vi "SPI Configuration Main.vi"() -> ()   [LabVIEW 2014, in "SPI Configuration Tool.lvlib"]
doc: "This is the main VI for the configuration editor."
uses:
  SPI Configuration Tool.lvlib
  Controls/StateCluster.ctl
  <vilib>/NI/Configuration Framework/Repository/NISE_CEF_Repository.lvclass
  <vilib>/NI/Configuration Framework/Node/NodeRef.ctl
  <vilib>/NI/Configuration Framework/Node/NISE_CEF_Node.lvclass
  <vilib>/NI/Configuration Framework/Node/UserEventRef.ctl
  <vilib>/NI/Configuration Framework/Controls/EventCluster.ctl
  <vilib>/Utility/error.llb/DialogType.ctl
  <vilib>/NI/Configuration Framework/hierarchy repo/NISE_CEF_HierarchyRepo.lvclass
  Classes/My System/My System.lvclass
  Controls/AddMessage.ctl
  Controls/MoveMessage.ctl
  Classes/RIO Target/RIO Target.lvclass
  <vilib>/NI/AMC/Read Termination Message.vi
  <vilib>/NI/AMC/Create Single Message.vi
  <vilib>/NI/AMC/Update Message Routing Info.vi
  <vilib>/NI/AMC/Globals.vi
  <vilib>/NI/AMC/Send Message.vi
  <vilib>/NI/AMC/AMC.lvlib
  <vilib>/NI/Configuration Framework/NISE_CEF_TreeControl.lvlib
  <vilib>/NI/Configuration Framework/serializable configuration/NISE_CEF_serializable configuration.lvclass
panel:
  in  "View":string(tree)
  in  "Exit":bool
  # "SPI Inteface Generation"
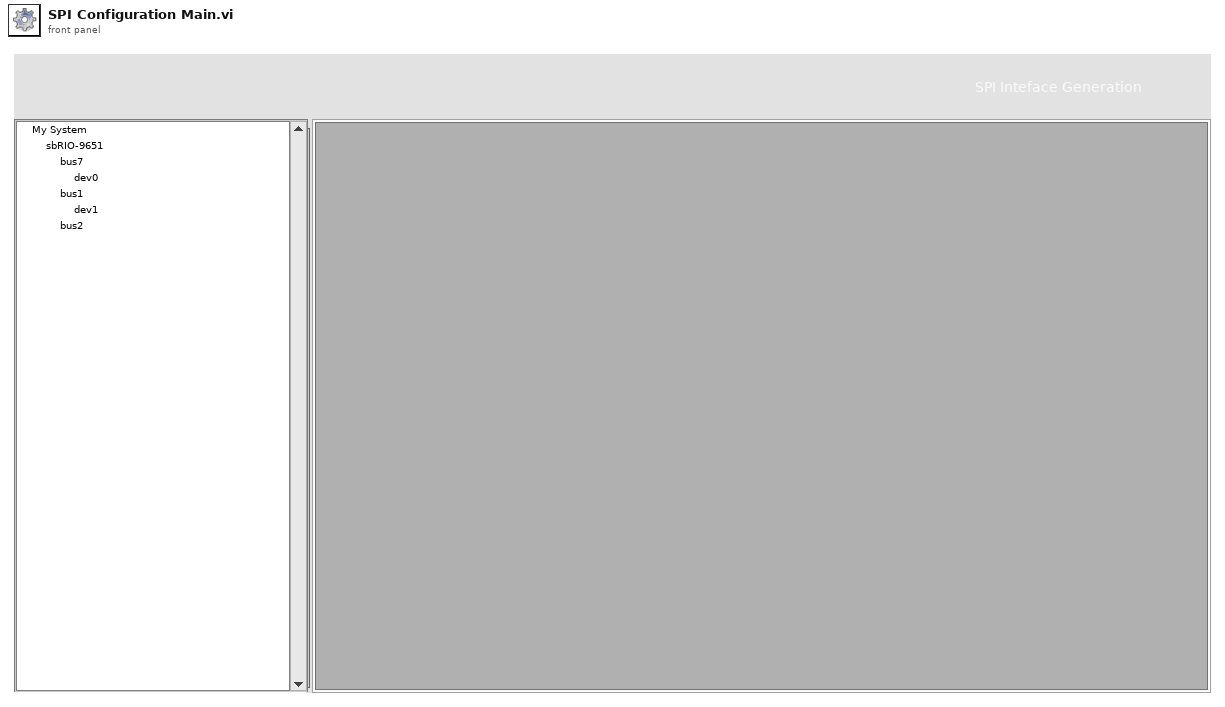
[diagram p1: front panel]
types:
  T1 = typedef "SPI Configuration Tool.lvlib/StateCluster.ctl" = cluster{"repository":refnum<class "NISE_CEF_Repository.lvclass">, "root":T2, "unsaved changes":bool, "current path":path, "user event ref":T3, "glyph path":path, "classes path":path}
  T2 = typedef "NISE_CEF_Node.lvclass/NodeRef.ctl" = refnum<data-value>
  T3 = typedef "NISE_CEF_Node.lvclass/UserEventRef.ctl" = refnum<user-event>
  T4 = typedef "AMC.lvlib/Message Queue.ctl" = refnum<queue>
  T5 = typedef "SPI Configuration Tool.lvlib/AddMessage.ctl" = cluster{"node type":string, "to add to":string}
  T6 = typedef "SPI Configuration Tool.lvlib/MoveMessage.ctl" = cluster{"node ref":T2, "new parent":T2}
  T7 = enum32{"Invalid", "Standard", "Closed", "Hidden", "Minimized", "Maximized"}
  T8 = typedef "NISE_CEF_TreeControl.lvlib/EventCluster.ctl" = cluster{"command":string, "data":string}
  T9 = typedef "SPI Configuration Tool.lvlib/FilePaths.ctl" = cluster{"glyphs":path, "classes":path}
  T10 = typedef "DialogType.ctl" = u16
  T11 = typedef "NISE_CEF_Node.lvclass/Summary.ctl" = cluster{"ID":string, "parent ID":string, "node type":string, "text":string, "additional text":string, "glyph":string, "depth":i32, "glyph overlay":string}
  T12 = typedef "LVPoint32TypeDef.ctl" = cluster{"Horizontal":i32, "Vertical":i32}
  T13 = cluster{"data name":string, "drag data":variant}[]
  T14 = typedef "NISE_CEF_Node.lvclass/NodeMenuOptions.ctl" = cluster{"removable":bool, "movable":bool, "duplicate":bool}
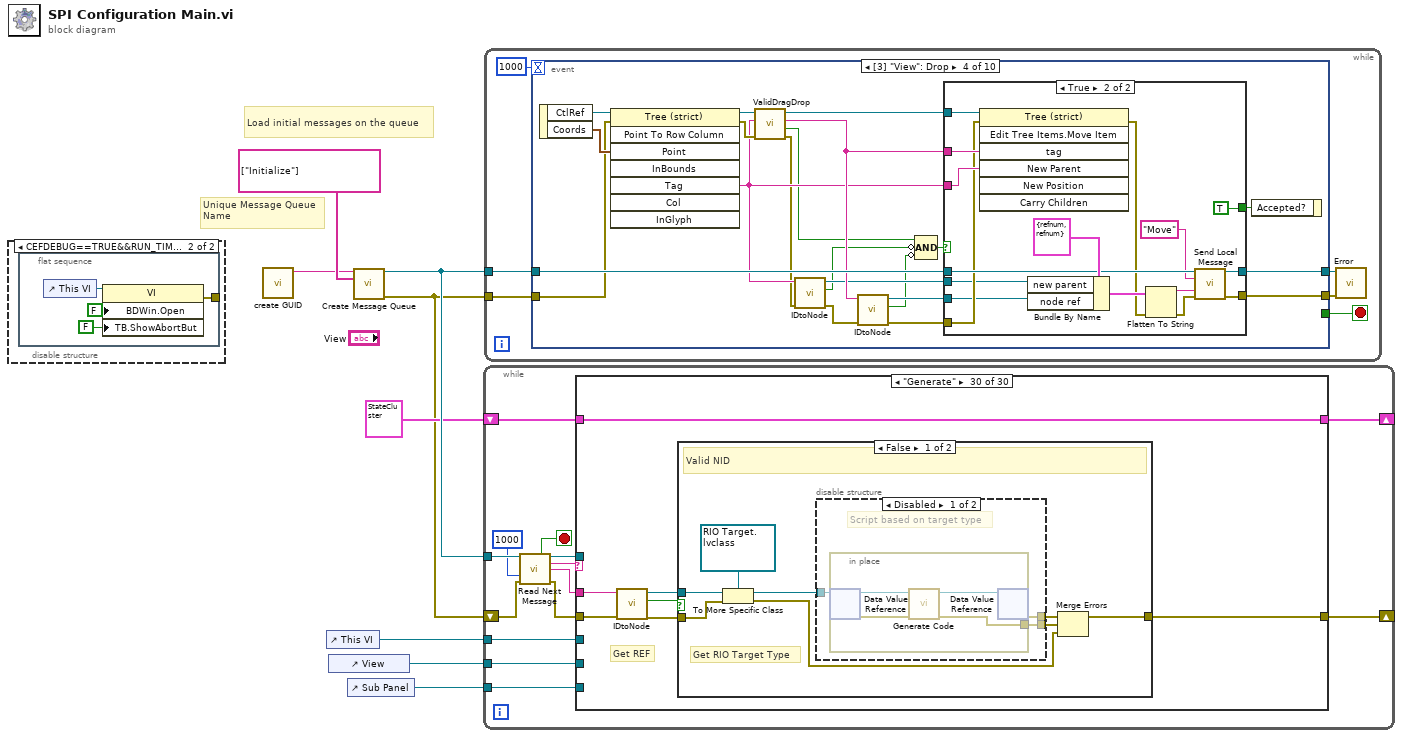
[diagram p0: block diagram]
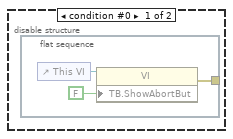
[diagram p2: hidden frame]
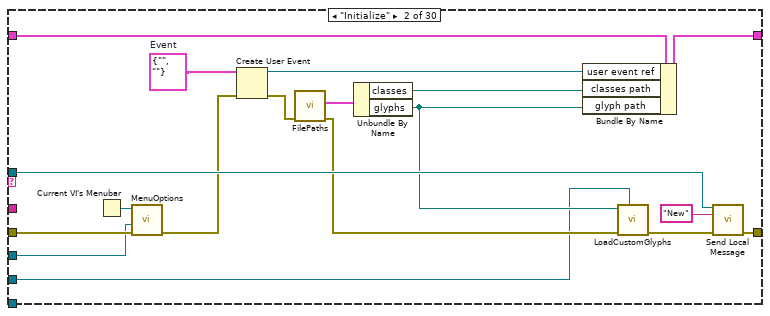
[diagram p4: hidden frame]
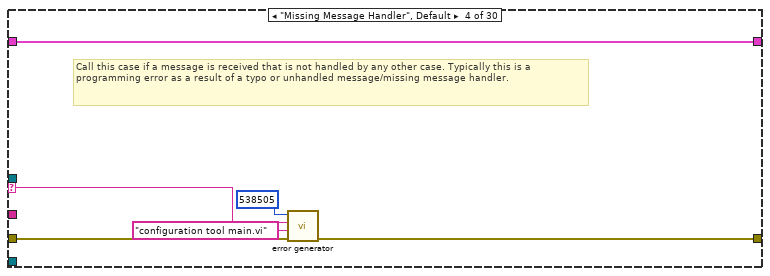
[diagram p6: hidden frame]
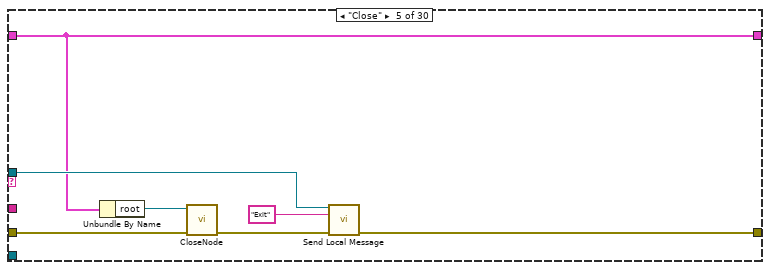
[diagram p7: hidden frame]
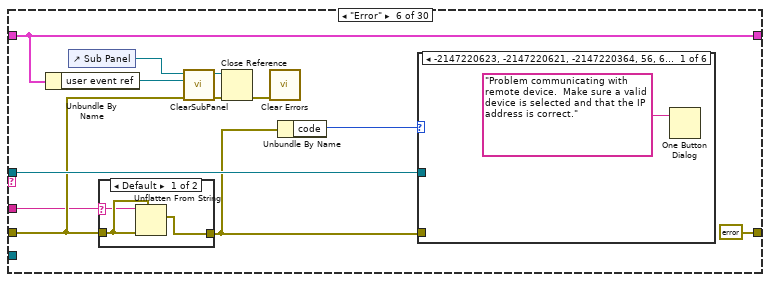
[diagram p8: hidden frame]
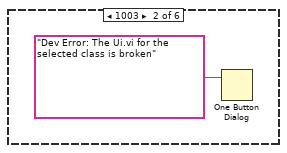
[diagram p10: hidden frame]
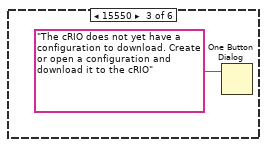
[diagram p11: hidden frame]
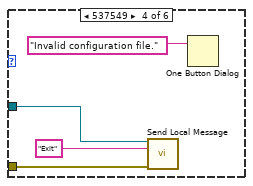
[diagram p12: hidden frame]
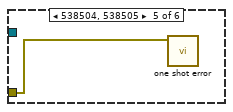
[diagram p13: hidden frame]
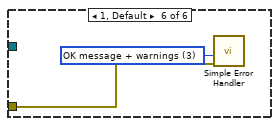
[diagram p14: hidden frame]
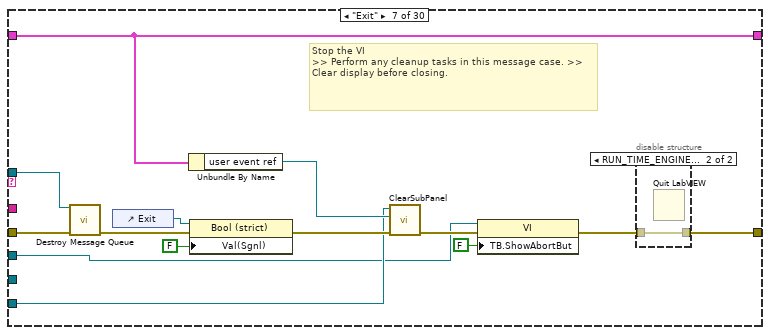
[diagram p15: hidden frame]
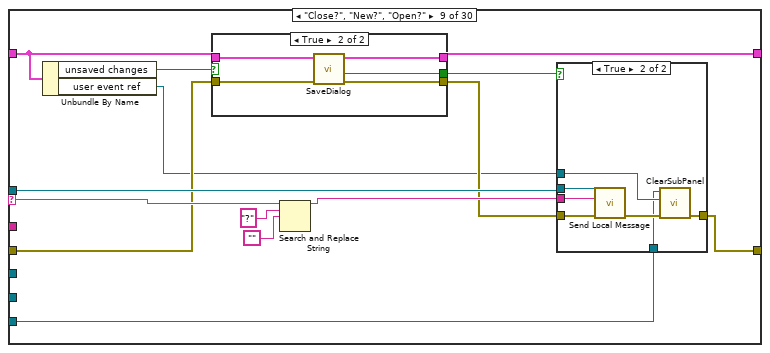
[diagram p18: hidden frame]
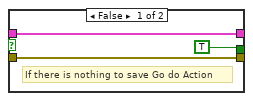
[diagram p19: hidden frame]
diagram:
  # "Unique Message Queue Name"
  # "Load initial messages on the queue"
  n1 = disable-structure shown="CEFDEBUG==TRUE&&RUN_TIME_ENGINE==False" {
    frame condition #0 {
      n2 = flat-sequence {
        tunnel: [w9] -> _
        frame #0 {
          n3 = control-ref of="This VI"() -> (w10:refnum<vi>)
          n4 = property class="VI"(reference=w10, "TB.ShowAbortBut"=FALSE ("Tool Bar:Show Abort Button")) -> (error out=w9:errorcluster)  [unwired: 1 in, 1 out]
        }
      }
    }
    frame condition #1 (active) {
      n5 = flat-sequence {
        tunnel: [w14] -> _
        frame #0 {
          n6 = control-ref of="This VI"() -> (w15:refnum<vi>)
          n7 = property class="VI"(reference=w15, "BDWin.Open"=FALSE ("Block Diagram Window:Open"), "TB.ShowAbortBut"=FALSE ("Tool Bar:Show Abort Button")) -> (error out=w14:errorcluster)  [unwired: 1 in, 1 out]
        }
      }
    }
  }
  n8 = call <vilib>:"create GUID.vi"() -> ("uuid"=w2:string)  [unwired: 10 in, 1 out]
  n9 = control-ref of="This VI"() -> (w4:refnum<vi>)
  n10 = control-ref of="View"() -> (w3:refnum<vi>)
  n11 = control-ref of="Sub Panel"() -> (w1:refnum<vi>)
  n12 = call <vilib>:"Create Message Queue.vi"("message queue name"=w2, "initial message names"=string[] ["Initialize"]) -> ("message queue out"=w7:T4, "error out"=w5:errorcluster)  [unwired: 12 in]
  n13 = while "Message Processor" {
    shift-right: [w25] -> _
    shift-left: w5 -> [w24]
    tunnel: w7 -> [w23]
    shift-right: [w21] -> _
    shift-left: T1 {"repository"=refnum, "root"=refnum, "unsaved changes"=FALSE, "current path"=path "", "user event ref"=refnum, "glyph path"=path "", "classes path"=path ""} -> [w20]
    tunnel: w4 -> [w18]
    tunnel: w3 -> [w17]
    tunnel: w1 -> [w16]
    stop <- w29 stop-if-true
    n14 = call <vilib>:"Read Next Message.vi"("message queue in"=w23, "timeout (1 ms)"=1000, "error in"=w24) -> ("exit process?"=w29:bool, "message queue out"=w19:T4, "message name"=w28:string, "message value"=w27:string, "error out"=w26:errorcluster)  [unwired: 5 in, 3 out]
    n15 = case shown="\"Generate\"" w28 {
      selector: w28 -> [_ _ _ w54 _ _ _ _ w118 _ _ _ _ _ _ _ _ _ _ w371 _ _ _ _ _ _ _ _ _ _]
      tunnel: w27 -> [_ _ _ _ _ w65 _ _ _ _ _ _ _ w240 w272 _ w300 w337 w351 w369 w411 w435 _ _ w478 w500 _ _ _ w516]
      tunnel: w26 -> [w31 w49 w51 w56 w59 w68 w104 w108 w111 w155 w166 w206 w232 w247 w273 w290 w301 w330 w350 w374 w413 w434 w459 w468 w477 w498 w503 w505 w510 w517]
      tunnel: [w31 w45 w51 w55 w63 errorcluster {"status"=FALSE, "code"=0, "source"=""} ("error out") w97 w108 w122 w146 w162 w210 w234 w244 w260 w290 w304 w321 w354 w377 w417 w431 w454 w463 w474 w493 w503 w504 w509 w512] -> w25
      tunnel: [w30 w40 w50 w57 w61 w73 w96 w107 w113 w159 w167 w213 w233 w241 w269 w289 w307 w323 w347 w378 w415 w428 w461 w467 w472 w489 w502 w507 w511 w518] -> w21
      tunnel: w20 -> [w30 w41 w50 w57 w61 w73 w96 w107 w114 w158 w168 w208 w231 w242 w270 w289 w303 w328 w355 w378 w416 w436 w461 w467 w472 w501 w502 w507 w511 w518]
      tunnel: w19 -> [_ w44 _ _ w62 w76 w103 _ w121 w160 w164 w209 _ w243 w265 _ w291 w320 _ w372 _ _ _ _ w473 w492 _ _ _ _]
      tunnel: w18 -> [_ w32 _ _ _ _ w92 _ _ _ _ _ _ _ _ _ _ _ _ _ _ _ w446 _ _ _ _ _ _ _]
      tunnel: w17 -> [_ w33 _ _ _ _ _ _ _ _ _ _ _ _ _ _ _ w324 w348 w367 w408 w429 w447 _ _ _ _ _ _ _]
      tunnel: w16 -> [_ _ _ _ _ _ w94 _ w109 _ _ _ _ _ _ _ _ _ _ _ _ _ w444 w462 w469 _ _ _ _ _]
      frame "------------Generic Operations------------" {
        # "Dummy case to add a seperation in the Case Structure menu"
      }
      frame "Initialize" {
        w35 = T8 {"command"="", "data"=""}  # Event
        n16 = Current VI's Menubar() -> (w48:refnum<k9>)
        n17 = call "MenuOptions.vi"("error in"=w49, "VI ref"=w32, "menu ref in"=w48) -> ("error out"=w39:errorcluster)  [unwired: 7 in, 1 out]
        n18 = Create User Event(user event datatype=w35, error in=w39) -> (user event=w34:refnum<user-event>, error out=w38:errorcluster)
        n19 = call "FilePaths.vi"("error in"=w38) -> ("error out"=w43:errorcluster, "paths"=w42:T9)  [unwired: 9 in]
        n20 = Unbundle By Name(w42) -> ("classes"=w37:path, "glyphs"=w36:path)
        n21 = Bundle By Name(cluster=w41, "user event ref"=w34, "classes path"=w37, "glyph path"=w36) -> (w40:T1)
        n22 = call <vilib>:"LoadCustomGlyphs.vi"("tree ref"=w33, "error in"=w43, "glyph directory"=w36) -> ("error out"=w46:errorcluster)  [unwired: 8 in]
        n23 = call <vilib>:"Send Local Message.vi"("message queue in"=w44, "message name"="New" ("Message Name"), "error in"=w46) -> ("error out"=w45:errorcluster)  [unwired: 10 in, 2 out]
      }
      frame "", "Idle" {
      }
      frame "Missing Message Handler", Default {
        # "Call this case if a message is received that is not handled by any other case. Typically this is a programming error as a result of a typo or unhandled message/missing message handler."
        n24 = call <vilib>:"error generator.vi"("error in"=w56, "source"="configuration tool main.vi", "append error message"=w54, "error code (0)"=538505) -> ("error out"=w55:errorcluster)  [unwired: 5 in]
      }
      frame "Close" {
        n25 = Unbundle By Name(w61) -> ("root"=w60:T2)
        n26 = call <vilib>:"CloseNode.vi"("error in"=w59, "node ref"=w60) -> ("error out"=w58:errorcluster)  [unwired: 9 in]
        n27 = call <vilib>:"Send Local Message.vi"("message queue in"=w62, "message name"="Exit", "error in"=w58) -> ("error out"=w63:errorcluster)  [unwired: 10 in, 2 out]
      }
      frame "Error" {
        n28 = Unbundle By Name(w73) -> ("user event ref"=w71:T3)
        n29 = control-ref of="Sub Panel"() -> (w72:refnum<vi>)
        n30 = case shown="Default" w65 {
          selector: w65 -> [w78 _]
          tunnel: w68 -> [w79 w80]
          tunnel: [w77 w80] -> w67
          frame Default {
            n31 = Unflatten From String(type=w79, binary string=w78, error in (no error)=w79) -> (value=w77:errorcluster)  [unwired: 2 in, 2 out]
          }
          frame "" {
          }
        }
        n32 = call <vilib>:"ClearSubPanel.vi"("error in"=w68, "user event ref"=w71, "sub panel ref in"=w72) -> ("error out"=w70:errorcluster, "sub panel ref out"=w69:refnum<vi>)  [unwired: 7 in]
        n33 = Close Reference(reference=w69, error in (no error)=w70) -> (error out=w66:errorcluster)
        n34 = call <vilib>:"Clear Errors.vi"("error in (no error)"=w66) -> ()  [unwired: 5 in, 2 out]
        n35 = Unbundle By Name(w67) -> ("code"=w74:i32)
        n36 = case shown="-2147220623, -2147220621, -2147220364, 56, 63" w74 {
          tunnel: w76 -> [_ _ _ w86 _ _]
          tunnel: w67 -> [_ _ _ w85 w88 w90]
          frame -2147220623, -2147220621, -2147220364, 56, 63 {
            n37 = One Button Dialog(message="Problem communicating with remote device.  Make sure a valid device is selected and that the IP address is correct.") -> ()  [unwired: 1 in, 1 out]
          }
          frame 1003 {
            n38 = One Button Dialog(message="Dev Error: The Ui.vi for the selected class is broken") -> ()  [unwired: 1 in, 1 out]
          }
          frame 15550 {
            n39 = One Button Dialog(message="The cRIO does not yet have a configuration to download. Create or open a configuration and download it to the cRIO") -> ()  [unwired: 1 in, 1 out]
          }
          frame 537549 {
            n40 = call <vilib>:"Send Local Message.vi"("message queue in"=w86, "message name"="Exit", "error in"=w85) -> ()  [unwired: 10 in, 3 out]
            n41 = One Button Dialog(message="Invalid configuration file.") -> ()  [unwired: 1 in, 1 out]
          }
          frame 538504, 538505 {
            n42 = call <vilib>:"one shot error.vi"("error in"=w88) -> ()  [unwired: 11 in]
          }
          frame 1, Default {
            w89 = T10 3 items=["no dialog", "OK message", "continue or stop message", "OK message + warnings", "continue/stop + warnings"] ("type of dialog (OK msg:1)")
            n43 = call <vilib>:"Simple Error Handler.vi"("type of dialog (OK msg:1)"=w89, "error in (no error)"=w90) -> ()  [unwired: 8 out]
          }
        }
      }
      frame "Exit" {
        # "Stop the VI                                                                             >> Perform any cleanup tasks in this message case. >> Clear display before closing."
        n44 = call <vilib>:"Destroy Message Queue.vi"("message queue in"=w103, "error in"=w104) -> ("error out"=w100:errorcluster)  [unwired: 11 in, 2 out]
        n45 = control-ref of="Exit"() -> (w102:refnum<vi>)
        n46 = Unbundle By Name(w96) -> ("user event ref"=w95:T3)
        n47 = property class="Bool (strict)"(reference=w102, error in=w100, "Val(Sgnl)"=FALSE ("Exit")) -> (error out=w99:errorcluster)  [unwired: 1 out]
        n48 = call <vilib>:"ClearSubPanel.vi"("error in"=w99, "user event ref"=w95, "sub panel ref in"=w94) -> ("error out"=w98:errorcluster)  [unwired: 7 in, 1 out]
        n49 = property class="VI"(reference=w92, error in=w98, "TB.ShowAbortBut"=FALSE ("Tool Bar:Show Abort Button")) -> (error out=w93:errorcluster)  [unwired: 1 out]
        n50 = disable-structure shown="RUN_TIME_ENGINE==True" {
          disable-tunnel: [w105 w106] -> w97
          disable-tunnel: w93 -> [w105 w106]
          frame condition #0 (active) {
          }
          frame condition #1 {
            n51 = Quit LabVIEW() -> ()  [unwired: 1 in]
          }
        }
      }
      frame "------------Menu Operations--------------" {
        # "Dummy case to add a seperation in the Case Structure menu"
      }
      frame "Close?", "New?", "Open?" {
        n52 = Unbundle By Name(w114) -> ("unsaved changes"=w116:bool, "user event ref"=w110:T3)
        n53 = case shown="True" w116 {
          tunnel: [TRUE ("SaveFlag") w130] -> w115
          tunnel: w114 -> [w124 w129]
          tunnel: [w124 w128] -> w113
          tunnel: w111 -> [w123 w127]
          tunnel: [w123 w126] -> w112
          frame False {
            # "If there is nothing to save Go do Action"
          }
          frame True {
            n54 = call "SaveDialog.vi"("error in"=w127, "state in"=w129) -> ("error out"=w126:errorcluster, "new"=w130:bool, "state out"=w128:T1)  [unwired: 7 in]
          }
        }
        n55 = Search and Replace String(input string=w118, search string="?", replace string="") -> (result string=w117:string)  [unwired: 5 in, 3 out]
        n56 = case shown="True" w115 {
          tunnel: w112 -> [w131 w138]
          tunnel: [w131 w134] -> w122
          tunnel: w121 -> [_ w137]
          tunnel: w117 -> [_ w136]
          tunnel: w110 -> [_ w133]
          tunnel: w109 -> [_ w132]
          frame False {
          }
          frame True {
            n57 = call <vilib>:"Send Local Message.vi"("message queue in"=w137, "message name"=w136, "error in"=w138) -> ("error out"=w135:errorcluster)  [unwired: 10 in, 2 out]
            n58 = call <vilib>:"ClearSubPanel.vi"("error in"=w135, "user event ref"=w133, "sub panel ref in"=w132) -> ("error out"=w134:errorcluster)  [unwired: 7 in, 1 out]
          }
        }
      }
      frame "New" {
        n59 = Unbundle By Name(w158) -> ("classes path"=w157:path)
        n60 = call-dynamic "Initialize.vi"("error in"=w155, "path"=w157, "repository in"=refnum<class "NISE_CEF_HierarchyRepo.lvclass"> refnum ("NISE_CEF_HierarchyRepo.lvclass")) -> ("error out"=w156:errorcluster, "repository out"=w149:refnum<class "NISE_CEF_HierarchyRepo.lvclass">)  [unwired: 7 in]
        n61 = call-dynamic "Initialize.vi"("error in"=w156, "node in"=refnum<class "My System.lvclass"> refnum ("My System.lvclass")) -> ("error out"=w143:errorcluster, "data value reference"=w144:T2)  [unwired: 7 in, 1 out]
        n62 = call <vilib>:"NodetoID.vi"("error in"=w143, "node ref"=w144) -> ("error out"=w142:errorcluster, "ID"=w140:string)  [unwired: 8 in]
        n63 = call <vilib>:"Send Local Message.vi"("message queue in"=w160, "message name"="PopulateTree", "error in"=w142) -> ("message queue out"=w145:T4, "error out"=w151:errorcluster)  [unwired: 10 in, 1 out]
        n64 = Current VI's Menubar() -> (w150:refnum<k9>)
        n65 = call <vilib>:"NewMenu.vi"("error in"=w151, "menu ref in"=w150, "NISE_CEF_Repository in"=w149) -> ("error out"=w147:errorcluster, "NISE_CEF_Repository out"=w148:refnum<class "NISE_CEF_HierarchyRepo.lvclass">)  [unwired: 6 in, 1 out]
        n66 = Bundle By Name(cluster=w158, "current path"=path "", "unsaved changes"=FALSE, "repository"=w148, "root"=w144) -> (w159:T1)
        n67 = call <vilib>:"Send Local Message.vi"("message queue in"=w145, "message name"="ActivateNode", "message value"=w140, "error in"=w147) -> ("error out"=w146:errorcluster)  [unwired: 9 in, 2 out]
      }
      frame "Open" {
        n68 = in-place {
          in-place-border: w166 -> [w174]
          in-place-border: [w173] -> w163
          n69 = in-place-cluster #1(w168) -> ("current path"=w170:path, "repository"=w182:refnum<class "NISE_CEF_Repository.lvclass">, "root"=w178:T2)  [unwired: 1 out]
          n70 = call "generate default path.vi"("current file path"=w170) -> ("browse path"=w169:path)  [unwired: 10 in]
          n71 = call "FileDialog.vi"("error in"=w174, "start path"=w169) -> ("error out"=w175:errorcluster, "cancelled"=w176:bool, "selected path"=w172:path)  [unwired: 7 in]
          n72 = Compound Arithmetic op=OR(invert w176) -> (w177:bool)
          n73 = case shown="True" w177 {
            tunnel: w182 -> [w183 w195]
            tunnel: [w183 w193] -> w180
            tunnel: [w184 w191] -> w173
            tunnel: [w185 w190] -> w179
            tunnel: w172 -> [_ w188]
            tunnel: w175 -> [w184 w187]
            tunnel: w178 -> [w185 w186]
            frame False {
            }
            frame True {
              n74 = call-dynamic "Open.vi"("error in"=w187, "file path"=w188, "repository in"=w195) -> ("error out"=w192:errorcluster, "invalid?"=w189:bool, "repository out"=w194:refnum<class "NISE_CEF_Repository.lvclass">)  [unwired: 6 in]
              n75 = case shown="False" w189 {
                tunnel: w194 -> [w200 w203]
                tunnel: [w199 w203] -> w193
                tunnel: w192 -> [w198 w202]
                tunnel: [w197 w202] -> w191
                tunnel: [w196 w201] -> w190
                tunnel: w186 -> [_ w201]
                frame False {
                  n76 = call-dynamic "WriteTree.vi"("error in"=w198, "repository in"=w200) -> ("error out"=w197:errorcluster, "root"=w196:T2, "repository out"=w199:refnum<class "NISE_CEF_Repository.lvclass">)  [unwired: 7 in]
                }
                frame True {
                }
              }
            }
          }
          n77 = Select(t=w170, s=w173, f=w172) -> (s? t:f=w171:path)
          n78 = in-place-cluster #1("current path"=w171, "unsaved changes"=FALSE ("SaveFlag"), "repository"=w180, "root"=w179) -> (w167:T1)
        }
        n79 = call <vilib>:"Send Local Message.vi"("message queue in"=w164, "message name"="PopulateTree", "error in"=w163) -> ("error out"=w162:errorcluster)  [unwired: 10 in, 2 out]
      }
      frame "Save" {
        n80 = in-place {
          in-place-border: w206 -> [w218]
          in-place-border: [w217] -> w205
          in-place-border: [w215] -> w204
          n81 = in-place-cluster #2(w208) -> ("current path"=w216:path, "root"=w219:T2, "repository"=w220:refnum<class "NISE_CEF_Repository.lvclass">)
          n82 = Empty String/Path?(string/path=w216) -> (empty?=w215:bool)
          n83 = call-dynamic "ReadTree.vi"("error in"=w218, "root"=w219, "repository in"=w220) -> ("error out"=w217:errorcluster, "repository out"=w214:refnum<class "NISE_CEF_Repository.lvclass">)  [unwired: 7 in]
          n84 = in-place-cluster #2("current path"=w216, "root"=w219, "repository"=w214) -> (w207:T1)
        }
        n85 = case shown="True" w204 {
          tunnel: w207 -> [w224 w226]
          tunnel: [w223 w225] -> w213
          tunnel: [w222 w227] -> w211
          tunnel: w205 -> [w221 w228]
          frame False {
            n86 = call "Save.vi"("error in"=w221, "state in"=w224) -> ("error out"=w222:errorcluster, "state out"=w223:T1)  [unwired: 8 in]
          }
          frame True {
            # "Empty path use Dialog"
            n87 = call "SaveAs.vi"("error in"=w228, "state in"=w226) -> ("error out"=w227:errorcluster, "state out"=w225:T1)  [unwired: 7 in, 1 out]
          }
        }
        n88 = call <vilib>:"Send Local Message.vi"("message queue in"=w209, "message name"="PopulateTree", "error in"=w211) -> ("error out"=w210:errorcluster)  [unwired: 10 in, 2 out]
      }
      frame "SaveAs" {
        n89 = in-place {
          in-place-border: w232 -> [w236]
          in-place-border: [w235] -> w230
          n90 = in-place-cluster #3(w231) -> ("root"=w237:T2, "repository"=w239:refnum<class "NISE_CEF_Repository.lvclass">)
          n91 = call-dynamic "ReadTree.vi"("error in"=w236, "root"=w237, "repository in"=w239) -> ("error out"=w235:errorcluster, "repository out"=w238:refnum<class "NISE_CEF_Repository.lvclass">)  [unwired: 7 in]
          n92 = in-place-cluster #3("root"=w237, "repository"=w238) -> (w229:T1)
        }
        n93 = call "SaveAs.vi"("error in"=w230, "state in"=w229) -> ("error out"=w234:errorcluster, "state out"=w233:T1)  [unwired: 7 in, 1 out]
      }
      frame "Custom View" {
        n94 = in-place {
          in-place-border: w247 -> [w258]
          in-place-border: [w257] -> w245
          in-place-border: w240 -> [w248]
          n95 = in-place-cluster #4(w242) -> ("repository"=w252:refnum<class "NISE_CEF_Repository.lvclass">, "root"=w251:T2)
          n96 = call-dynamic "ReadTree.vi"("error in"=w258, "root"=w251, "repository in"=w252) -> ("error out"=w255:errorcluster, "repository out"=w254:refnum<class "NISE_CEF_Repository.lvclass">)  [unwired: 7 in]
          n97 = call-dynamic "CustomView.vi"("error in"=w255, "view name"=w248, "repository in"=w254) -> ("error out"=w256:errorcluster, "repository out"=w253:refnum<class "NISE_CEF_Repository.lvclass">)  [unwired: 7 in]
          n98 = call-dynamic "WriteTree.vi"("error in"=w256, "repository in"=w253) -> ("error out"=w257:errorcluster, "root"=w249:T2, "repository out"=w250:refnum<class "NISE_CEF_Repository.lvclass">)  [unwired: 7 in]
          n99 = in-place-cluster #4("repository"=w250, "root"=w249) -> (w241:T1)
        }
        n100 = call <vilib>:"Send Local Message.vi"("message queue in"=w243, "message name"="PopulateTree", "error in"=w245) -> ("error out"=w244:errorcluster)  [unwired: 10 in, 2 out]
      }
      frame "CustomFileMenu" {
        n101 = Unflatten From String(type=cluster{"ItemTag":string, string} {"ItemTag"="", ""} ("output cluster"), binary string=w272, error in (no error)=w273) -> (value=w259:cluster{"ItemTag":string, string}, error out=w268:errorcluster)  [unwired: 2 in, 1 out]
        n102 = Unbundle By Name(w270) -> ("repository"=w267:refnum<class "NISE_CEF_Repository.lvclass">)
        n103 = Unbundle(w259) -> ("ItemTag"=w264:string, w263:string)
        n104 = call-dynamic "HandleMenu.vi"("message queue"=w265, "error in"=w268, "Item Path"=w263, "ItemTag"=w264, "NISE_CEF_Repository in"=w267) -> ("error out"=w262:errorcluster, "handled?"=w261:bool, "NISE_CEF_Repository out"=w266:refnum<class "NISE_CEF_Repository.lvclass">)  [unwired: 4 in]
        n105 = case shown="False" w261 {
          tunnel: w262 -> [w277 w288]
          tunnel: [w278 w288] -> w260
          tunnel: w259 -> [w276 _]
          frame False {
            n106 = Unbundle(w276) -> ("ItemTag"=w275:string, w274:string)
            n107 = disable-structure shown="Default" {
              disable-tunnel: w277 -> [w284 w287]
              disable-tunnel: [w283 w287] -> w278
              disable-tunnel: w274 -> [w282 _]
              disable-tunnel: w275 -> [w281 _]
              frame condition #0 (active) {
                n108 = Concatenate Strings(w281, "::" ("string"), w282) -> (w280:string)
                n109 = call <vilib>:"error generator.vi"("error in"=w284, "source"="configuration tool main.vi", "append error message"=w280, "error code (0)"=538506) -> ("error out"=w283:errorcluster)  [unwired: 5 in]
              }
              frame condition #1 {
              }
            }
          }
          frame True {
          }
        }
        n110 = Bundle By Name(cluster=w270, "repository"=w266) -> (w269:T1)
      }
      frame "-------TreeControl Operations-----------" {
        # "Dummy case to add a seperation in the Case Structure menu"
      }
      frame "Select Target" {
        n111 = in-place {
          in-place-border: w301 -> [w311]
          in-place-border: w300 -> [w310]
          in-place-border: [w309] -> w297
          in-place-border: [w308] -> w298
          n112 = in-place-cluster #5(w303) -> ("repository"=w313:refnum<class "NISE_CEF_Repository.lvclass">)
          n113 = call-dynamic "GetClassPath.vi"("error in"=w311, "class name"=w310, "Repository in"=w313) -> ("error out"=w309:errorcluster, "class path"=w308:path, "Repository out"=w312:refnum<class "NISE_CEF_Repository.lvclass">)  [unwired: 6 in]
          n114 = in-place-cluster #5("repository"=w312) -> (w302:T1)
        }
        n115 = call <vilib>:"Get LV Class Default Value.vi"("error in (no error)"=w297, "class path"=w298) -> ("error out"=w296:errorcluster, "object"=w299:refnum<class>)  [unwired: 8 in]
        n116 = To More Specific Class(target class=refnum<class "NISE_CEF_Node.lvclass"> refnum ("Node.lvclass"), reference=w299, error in=w296) -> (specific class reference=w294:refnum<class "NISE_CEF_Node.lvclass">, error out=w293:errorcluster)
        n117 = call-dynamic "Initialize.vi"("error in"=w293, "node in"=w294) -> ("error out"=w292:errorcluster, "data value reference"=w306:T2)  [unwired: 7 in, 1 out]
        n118 = Bundle By Name(cluster=w302, "root"=w306) -> (w307:T1)
        n119 = call <vilib>:"Send Local Message.vi"("message queue in"=w291, "message name"="PopulateTree", "error in"=w292) -> ("error out"=w304:errorcluster)  [unwired: 10 in, 2 out]
      }
      frame "AddNode" {
        n120 = Unflatten From String(type=T5 {"node type"="", "to add to"=""} ("input cluster"), binary string=w337) -> (value=w335:T5)  [unwired: 3 in, 2 out]
        n121 = Unbundle By Name(w335) -> ("to add to"=w333:string, "node type"=w326:string)
        n122 = in-place {
          in-place-border: w330 -> [w343]
          in-place-border: [w342] -> w329
          in-place-border: w326 -> [w341]
          in-place-border: [w340] -> w325
          n123 = in-place-cluster #6(w328) -> ("repository"=w345:refnum<class "NISE_CEF_Repository.lvclass">)
          n124 = call-dynamic "GetClassPath.vi"("error in"=w343, "class name"=w341, "Repository in"=w345) -> ("error out"=w342:errorcluster, "class path"=w340:path, "Repository out"=w344:refnum<class "NISE_CEF_Repository.lvclass">)  [unwired: 6 in]
          n125 = in-place-cluster #6("repository"=w344) -> (w327:T1)
        }
        n126 = call <vilib>:"Get LV Class Default Value.vi"("error in (no error)"=w329, "class path"=w325) -> ("error out"=w338:errorcluster, "object"=w339:refnum<class>)  [unwired: 8 in]
        n127 = To More Specific Class(target class=refnum<class "NISE_CEF_Node.lvclass"> refnum ("Node.lvclass"), reference=w339, error in=w338) -> (specific class reference=w318:refnum<class "NISE_CEF_Node.lvclass">, error out=w332:errorcluster)
        n128 = call <vilib>:"AddNode.vi"("error in"=w332, "node in"=w318, "parent node ID"=w333) -> ("error out"=w331:errorcluster, "summary"=w316:T11[])  [unwired: 7 in]
        n129 = Index Array(array=w316) -> (element=w315:T11)  [unwired: 1 in]
        n130 = call <vilib>:"PopulateTreeSumary.vi"("error in"=w331, "array"=w316, "tree ref in"=w324) -> ("error out"=w317:errorcluster)  [unwired: 8 in]
        n131 = Bundle By Name(cluster=w327, "unsaved changes"=TRUE) -> (w323:T1)
        n132 = Unbundle By Name(w315) -> ("ID"=w314:string)
        n133 = call <vilib>:"Send Local Message.vi"("message queue in"=w320, "message name"="ActivateNode", "message value"=w314, "error in"=w317) -> ("error out"=w321:errorcluster)  [unwired: 9 in, 2 out]
        n134 = property on="View" class="Tree (strict)"("Value"=w314) -> ()  [unwired: 2 in, 2 out]
      }
      frame "Duplicate" {
        n135 = call <vilib>:"IDtoNode.vi"("error in"=w350, "ID"=w351) -> ("error out"=w352:errorcluster, "invalid Id"=w349:bool, "node ref"=w353:T2)  [unwired: 7 in]
        n136 = case shown="False" w349 {
          tunnel: [w364 w365] -> w354
          tunnel: w353 -> [w363 _]
          tunnel: w352 -> [w360 w365]
          tunnel: w348 -> [w356 _]
          frame False {
            n137 = call <vilib>:"DuplicateNode.vi"("same parent?"=TRUE ("s"), "error in"=w360, "node ref in"=w363) -> ("error out"=w361:errorcluster, "new node ref"=w362:T2)  [unwired: 7 in]
            n138 = call <vilib>:"Summary.vi"("error in"=w361, "node self ref"=w362) -> ("error out"=w358:errorcluster, "summary"=w357:T11[])  [unwired: 8 in]
            n139 = call <vilib>:"PopulateTreeSumary.vi"("error in"=w358, "array"=w357, "tree ref in"=w356) -> ("error out"=w364:errorcluster)  [unwired: 8 in]
          }
          frame True {
          }
        }
        n140 = Bundle By Name(cluster=w355, "unsaved changes"=TRUE) -> (w347:T1)
      }
      frame "CustomMenuAction" {
        # "Pass NID into parameters\nto use in other cases"
        n141 = Match Pattern(string=w369, regular expression=":") -> (before substring=w368:string, after substring=w366:string)  [unwired: 1 in, 2 out]
        n142 = call <vilib>:"IDtoNode.vi"("error in"=w374, "ID"=w366) -> ("error out"=w375:errorcluster, "invalid Id"=w373:bool, "node ref"=w376:T2)  [unwired: 7 in]
        n143 = case shown="False" w373 {
          tunnel: [w383 w407] -> w377
          tunnel: w376 -> [w379 _]
          tunnel: w375 -> [w386 w407]
          tunnel: w372 -> [w387 _]
          tunnel: w371 -> [_ _]
          tunnel: w368 -> [w384 _]
          tunnel: w367 -> [w381 _]
          tunnel: w366 -> [w380 _]
          frame False {
            n144 = in-place {
              in-place-border: w387 -> [w405]
              in-place-border: w386 -> [w403]
              in-place-border: [w402] -> w382
              in-place-border: [w401] -> w385
              in-place-border: w384 -> [w400]
              in-place-border: w381 -> [w399]
              in-place-border: w380 -> [w398]
              n145 = in-place-dvr #7(w379) -> (w406:refnum<class "NISE_CEF_Node.lvclass">)  [unwired: 1 out]
              n146 = call-dynamic "MenuHandler.vi"("tree control"=w399, "main message queue"=w405, "error in"=w403, "parameters"=w398, "menu string"=w400, "NISE_CEF_Node in"=w406) -> ("error out"=w402:errorcluster, "Unhandled"=w401:bool, "NISE_CEF_Node out"=w404:refnum<class "NISE_CEF_Node.lvclass">)  [unwired: 2 in, 1 out]
              n147 = in-place-dvr #7(w404) -> ()  [unwired: 2 out]
            }
            n148 = case shown="False" w385 {
              tunnel: w384 -> [_ w389]
              tunnel: [w388 w390] -> w383
              tunnel: w382 -> [w388 w391]
              frame False {
              }
              frame True {
                n149 = disable-structure shown="CEFDEBUG==TRUE" {
                  disable-tunnel: w391 -> [w394 w397]
                  disable-tunnel: [w393 w397] -> w390
                  disable-tunnel: w389 -> [w392 _]
                  frame condition #0 (active) {
                    n150 = call <vilib>:"error generator.vi"("error in"=w394, "source"="configuration tool main.vi", "append error message"=w392, "error code (0)"=538506) -> ("error out"=w393:errorcluster)  [unwired: 5 in]
                  }
                  frame condition #1 {
                  }
                }
              }
            }
          }
          frame True {
          }
        }
      }
      frame "RefreshNode" {
        # "Refreshes the node in the Tree               Sets the save flag to true                       This case can be called from the UIs of the nodes"
        n151 = call <vilib>:"IDtoNode.vi"("error in"=w413, "ID"=w411) -> ("error out"=w412:errorcluster, "invalid Id"=w409:bool, "node ref"=w410:T2)  [unwired: 7 in]
        n152 = case shown="False" w409 {
          tunnel: [w424 w426] -> w417
          tunnel: w412 -> [w420 w426]
          tunnel: w410 -> [w419 _]
          tunnel: w408 -> [w418 _]
          frame False {
            n153 = call <vilib>:"Summary.vi"("error in"=w420, "node self ref"=w419) -> ("error out"=w422:errorcluster, "summary"=w421:T11[])  [unwired: 8 in]
            n154 = call <vilib>:"RefreshSubTree.vi"("error in"=w422, "node information"=w421, "tree ref in"=w418) -> ("error out"=w425:errorcluster, "tree ref out"=w423:refnum<vi>)  [unwired: 7 in]
            n155 = Close Reference(reference=w423, error in (no error)=w425) -> (error out=w424:errorcluster)
          }
          frame True {
          }
        }
        n156 = Bundle By Name(cluster=w416, "unsaved changes"=TRUE ("SaveFlag")) -> (w415:T1)
      }
      frame "RemoveNode" {
        n157 = call <vilib>:"IDtoNode.vi"("error in"=w434, "ID"=w435) -> ("error out"=w433:errorcluster, "invalid Id"=w430:bool, "node ref"=w432:T2)  [unwired: 7 in]
        n158 = case shown="False" w430 {
          tunnel: w433 -> [w442 w443]
          tunnel: w432 -> [w441 _]
          tunnel: [w438 w443] -> w431
          tunnel: w429 -> [w437 _]
          frame False {
            n159 = call <vilib>:"RemoveNode.vi"("error in"=w442, "node"=w441) -> ("error out"=w439:errorcluster, "node ID"=w440:string)  [unwired: 8 in]
            n160 = call <vilib>:"ClearTreeNode.vi"("error in"=w439, "tag"=w440, "tree reference"=w437) -> ("error out"=w438:errorcluster)  [unwired: 8 in]
          }
          frame True {
          }
        }
        n161 = Bundle By Name(cluster=w436, "unsaved changes"=TRUE) -> (w428:T1)
      }
      frame "PopulateTree" {
        n162 = Unbundle By Name(w461) -> ("current path"=w452:path, "user event ref"=w453:T3, "root"=w457:T2)
        n163 = call <vilib>:"Summary.vi"("error in"=w459, "depth"=0 ("Depth"), "node self ref"=w457) -> ("error out"=w458:errorcluster, "summary"=w460:T11[])  [unwired: 7 in]
        n164 = call <vilib>:"Check if File or Folder Exists.vi"("path"=w452) -> ("file or folder exists?"=w450:bool, "dup path"=w451:path)  [unwired: 8 in, 1 out]
        n165 = Strip Path(path=w451) -> (name=w449:string)  [unwired: 1 out]
        n166 = call <vilib>:"RefreshEntireTree.vi"("calling VI in"=w446, "error in"=w458, "array"=w460, "tree ref in"=w447) -> ("error out"=w455:errorcluster)  [unwired: 7 in]
        n167 = Select(t=w449, s=w450, f="Advanced Configurator Sample Project") -> (s? t:f=w445:string)
        n168 = property class="VI"(reference=w446, "Front Panel.Title"=w445) -> ()  [unwired: 1 in, 2 out]
        n169 = call <vilib>:"ClearSubPanel.vi"("error in"=w455, "user event ref"=w453, "sub panel ref in"=w444) -> ("error out"=w454:errorcluster)  [unwired: 7 in, 1 out]
      }
      frame "CleansubPanel" {
        n170 = Unbundle By Name(w467) -> ("user event ref"=w466:T3)
        n171 = call <vilib>:"ClearSubPanel.vi"("error in"=w468, "user event ref"=w466, "sub panel ref in"=w462) -> ("error out"=w465:errorcluster, "sub panel ref out"=w464:refnum<vi>)  [unwired: 7 in]
        n172 = Close Reference(reference=w464, error in (no error)=w465) -> (error out=w463:errorcluster)
      }
      frame "ActivateNode" {
        n173 = Unbundle By Name(w472) -> ("user event ref"=w471:T3)
        n174 = call <vilib>:"IDtoNode.vi"("error in"=w477, "ID"=w478) -> ("error out"=w470:errorcluster, "invalid Id"=w476:bool, "node ref"=w475:T2)  [unwired: 7 in]
        n175 = case shown="False" w476 {
          tunnel: w475 -> [w485 _]
          tunnel: [w486 w487] -> w474
          tunnel: w470 -> [w483 w487]
          tunnel: w473 -> [w481 _]
          tunnel: w471 -> [w482 _]
          tunnel: w469 -> [w479 _]
          frame False {
            n176 = call <vilib>:"ClearSubPanel.vi"("error in"=w483, "user event ref"=w482, "sub panel ref in"=w479) -> ("error out"=w484:errorcluster, "sub panel ref out"=w480:refnum<vi>)  [unwired: 7 in]
            n177 = call <vilib>:"LoadNodeUI.vi"("user event out"=w482, "error in"=w484, "sub panel ref in"=w480, "main queue"=w481, "node"=w485) -> ("error out"=w486:errorcluster)  [unwired: 6 in]
          }
          frame True {
          }
        }
      }
      frame "Move" {
        n178 = Unflatten From String(type=T6 {"node ref"=refnum, "new parent"=refnum} ("Cluster"), binary string=w500, error in (no error)=w498) -> (value=w497:T6, error out=w496:errorcluster)  [unwired: 2 in, 1 out]
        n179 = Unbundle By Name(w497) -> ("node ref"=w491:T2, "new parent"=w490:T2)
        n180 = call <vilib>:"MoveNode.vi"("error in"=w496, "new parent"=w490, "node"=w491) -> ("error out"=w494:errorcluster)  [unwired: 8 in]
        n181 = Bundle By Name(cluster=w501, "unsaved changes"=TRUE) -> (w489:T1)
        n182 = call <vilib>:"Send Local Message.vi"("message queue in"=w492, "message name"="PopulateTree", "error in"=w494) -> ("error out"=w493:errorcluster)  [unwired: 10 in, 2 out]
      }
      frame "-------Custom SPI Operations-----------" {
      }
      frame "Hide Front Panel" {
        n183 = property class="VI"(error in=w505, "FP.State"=T7."Hidden" ("Front Panel Window:State")) -> (error out=w504:errorcluster)  [unwired: 1 in, 1 out]
      }
      frame "Show Front Panel" {
        n184 = property class="VI"(error in=w510, "FP.State"=T7."Standard" ("State")) -> (error out=w509:errorcluster)  [unwired: 1 in, 1 out]
      }
      frame "Generate" {
        # "Get REF"
        n185 = call <vilib>:"IDtoNode.vi"("error in"=w517, "ID"=w516) -> ("error out"=w514:errorcluster, "invalid Id"=w513:bool, "node ref"=w515:T2)  [unwired: 7 in]
        n186 = case shown="False" w513 {
          tunnel: w515 -> [w526 _]
          tunnel: w514 -> [w525 w535]
          tunnel: [w519 w535] -> w512
          frame False {
            # "Get RIO Target Type"
            # "Valid NID"
            n187 = To More Specific Class(target class=refnum<data-value> refnum ("data value reference"), reference=w526, error in=w525) -> (specific class reference=w523:refnum<data-value>, error out=w520:errorcluster)
            n188 = disable-structure shown="Disabled" {
              disable-tunnel: w523 -> [w529 _]
              disable-tunnel: [w528 _] -> w522
              disable-tunnel: [w527 _] -> w521
              frame Disabled {
                # "Script based on target type"
                n189 = in-place {
                  in-place-border: [w530] -> w527
                  n190 = in-place-dvr #8(w529) -> (w533:refnum<class "RIO Target.lvclass">, w531:errorcluster)
                  n191 = call-dynamic "Generate Code.vi"("error in (no error)"=w531, "RIO Target in"=w533) -> ("error out"=w530:errorcluster, "RIO Target out"=w532:refnum<class "RIO Target.lvclass">)  [unwired: 8 in]
                  n192 = in-place-dvr #8(w532) -> (w528:errorcluster)  [unwired: 1 out]
                }
              }
              frame Enabled {
                n193 = Wait (ms)(milliseconds to wait=u32 2000) -> ()  [unwired: 1 out]
              }
            }
            n194 = Merge Errors(w522, w521, w520) -> (w519:errorcluster)
          }
          frame True {
            # "Invalid NID"
          }
        }
      }
    }
  }
  n195 = while "User Interface Event Handler" {
    tunnel: w7 -> [w540]
    tunnel: w5 -> [w536]
    stop <- w539 stop-if-true
    n196 = event shown="[3] \"View\": Drop" {
      selector: _ -> [_ _ _ _ _ _ _ _ _ _]
      dyn-events: _ -> [_ _ _ _ _ _ _ _ _ _]
      timeout: 1000 -> [_ _ _ _ _ _ _ _ _ _]
      tunnel: w540 -> [w543 w552 w577 w629 w657 w664 w693 w697 w707 w713]
      tunnel: [_ _ _ _ TRUE _ _ _ _ _] -> w539
      tunnel: [w543 w552 w574 w627 w653 w664 w690 w697 w705 w712] -> w538
      tunnel: [w542 w548 w573 w626 w654 w660 w689 w694 w703 w710] -> w537
      tunnel: w536 -> [w542 w551 w572 w628 w655 w663 w688 w696 w704 w711]
      event Timeout {
        # "Timeout code can be added here for autosave or Lock Screen"
        n197 = event-data() -> ()  [unwired: 1 in, 1 out]
      }
      event "View": Shortcut Menu Activation? {
        n198 = event-data() -> ("CtlRef"=w558:refnum<vi>, "Coords"=w557:T12, "MenuRef"=w554:refnum<k9>)  [unwired: 1 in]
        n199 = invoke class="Tree (strict)" method="Point To Row Column"(reference=w558, error in=w551, "Point"=w557) -> (error out=w550:errorcluster, "Tag"=w556:string)  [unwired: 5 in, 6 out]
        n200 = call <vilib>:"IDtoNode.vi"("error in"=w550, "ID"=w556) -> ("error out"=w546:errorcluster, "invalid Id"=w553:bool, "node ref"=w555:T2)  [unwired: 7 in]
        n201 = case shown="False" w553 {
          selector: w553 -> [_ w569]
          tunnel: w555 -> [w563 _]
          tunnel: w554 -> [w562 _]
          tunnel: [w561 _] -> w549
          tunnel: [w560 _] -> w547
          tunnel: w546 -> [w559 w570]
          tunnel: [w559 w570] -> w545
          tunnel: [_ w569] -> w544
          frame False {
            n202 = in-place {
              in-place-border: w562 -> [w566]
              in-place-border: [w564] -> w561
              n203 = in-place-dvr #9(w563) -> (w568:refnum<class "NISE_CEF_Node.lvclass">, w565:errorcluster)
              n204 = call-dynamic "ShortcutMenu.vi"("error in"=w565, "menu ref in"=w566, "node in"=w568) -> ("error out"=w564:errorcluster, "node out"=w567:refnum<class "NISE_CEF_Node.lvclass">)  [unwired: 6 in, 1 out]
              n205 = in-place-dvr #9(w567) -> (w560:errorcluster)  [unwired: 1 out]
            }
          }
          frame True {
          }
        }
        n206 = Merge Errors(w547, w549, w545) -> (w548:errorcluster)
        n207 = event-data("Discard?"=w544) -> ()  [unwired: 1 in, 1 out]
      }
      event "View": Shortcut Menu Selection (User) {
        n208 = event-data() -> ("ItemPath"=w576:string, "CtlRef"=w580:refnum<vi>, "Coords"=w581:T12)  [unwired: 1 in]
        n209 = invoke class="Tree (strict)" method="Point To Row Column"(reference=w580, error in=w572, "Point"=w581) -> (error out=w571:errorcluster, "Tag"=w575:string)  [unwired: 5 in, 6 out]
        n210 = Match Pattern(string=w576, regular expression=":") -> (before substring=w579:string, after substring=w578:string)  [unwired: 1 in, 2 out]
        n211 = case shown="\"Add\"" w579 {
          selector: w579 -> [w584 _ _ _]
          tunnel: w578 -> [_ _ _ w608]
          tunnel: w577 -> [w590 w597 w603 w610]
          tunnel: w575 -> [w586 w595 w601 w609]
          tunnel: [w587 w594 w600 w606] -> w574
          tunnel: [w588 w593 w598 w604] -> w573
          tunnel: w571 -> [w589 w592 w599 w605]
          frame Default {
            n212 = Concatenate Strings(w584, ":" ("string"), w586) -> (w583:string)
            n213 = call <vilib>:"Send Local Message.vi"("message queue in"=w590, "message name"="CustomMenuAction" ("Message Name"), "message value"=w583, "error in"=w589) -> ("message queue out"=w587:T4, "error out"=w588:errorcluster)  [unwired: 9 in, 1 out]
          }
          frame "Remove" {
            n214 = call <vilib>:"Send Local Message.vi"("message queue in"=w597, "message name"="RemoveNode" ("Message Name"), "message value"=w595, "error in"=w592) -> ("message queue out"=w594:T4, "error out"=w593:errorcluster)  [unwired: 9 in, 1 out]
          }
          frame "Duplicate" {
            n215 = call <vilib>:"Send Local Message.vi"("message queue in"=w603, "message name"="Duplicate" ("Message Name"), "message value"=w601, "error in"=w599) -> ("message queue out"=w600:T4, "error out"=w598:errorcluster)  [unwired: 9 in, 1 out]
          }
          frame "Add" {
            n216 = Bundle By Name(cluster=T5 {"node type"="", "to add to"=""} ("input cluster"), "node type"=w608, "to add to"=w609) -> (w611:T5)
            n217 = Flatten To String(anything=w611) -> (data string=w612:string)  [unwired: 3 in, 2 out]
            n218 = call <vilib>:"Send Local Message.vi"("message queue in"=w610, "message name"="AddNode" ("Message Name"), "message value"=w612, "error in"=w605) -> ("message queue out"=w606:T4, "error out"=w604:errorcluster)  [unwired: 9 in, 1 out]
          }
        }
      }
      event "View": Drop {
        n219 = event-data() -> ("CtlRef"=w632:refnum<vi>, "Coords"=w631:T12)  [unwired: 1 in]
        n220 = invoke class="Tree (strict)" method="Point To Row Column"(reference=w632, error in=w628, "Point"=w631) -> (reference out=w630:refnum<vi>, error out=w625:errorcluster, "Tag"=w622:string)  [unwired: 5 in, 5 out]
        n221 = call <vilib>:"ValidDragDrop.vi"("error in"=w625, "drag over"=w622, "tree ref in"=w630) -> ("error out"=w617:errorcluster, "accepted"=w620:bool, "drag"=w624:string, "tree ref out"=w634:refnum<vi>)  [unwired: 5 in]
        n222 = call <vilib>:"IDtoNode.vi"("error in"=w617, "ID"=w622) -> ("error out"=w618:errorcluster, "invalid Id"=w615:bool, "node ref"=w621:T2)  [unwired: 7 in]
        n223 = call <vilib>:"IDtoNode.vi"("error in"=w618, "ID"=w624) -> ("error out"=w616:errorcluster, "invalid Id"=w614:bool, "node ref"=w623:T2)  [unwired: 7 in]
        n224 = Compound Arithmetic op=AND(w620, invert w615, invert w614) -> (w619:bool)
        n225 = case shown="True" w619 {
          tunnel: w624 -> [_ w650]
          tunnel: w634 -> [_ w652]
          tunnel: [_ TRUE] -> w633
          tunnel: w622 -> [_ w648]
          tunnel: w629 -> [w636 w647]
          tunnel: [w636 w643] -> w627
          tunnel: [w635 w642] -> w626
          tunnel: w623 -> [_ w638]
          tunnel: w621 -> [_ w637]
          tunnel: w616 -> [w635 w639]
          frame False {
          }
          frame True {
            n226 = invoke class="Tree (strict)" method="Edit Tree Items.Move Item"(reference=w652, error in=w639, "tag"=w650, "New Parent"=w648) -> (error out=w640:errorcluster)  [unwired: 3 in, 6 out]
            n227 = Bundle By Name(cluster=T6 {"node ref"=refnum, "new parent"=refnum} ("Cluster"), "new parent"=w637, "node ref"=w638) -> (w646:T6)
            n228 = Flatten To String(anything=w646, error in (no error)=w640) -> (data string=w645:string, error out=w641:errorcluster)  [unwired: 2 in, 1 out]
            n229 = call <vilib>:"Send Local Message.vi"("message queue in"=w647, "message name"="Move", "message value"=w645, "error in"=w641) -> ("message queue out"=w643:T4, "error out"=w642:errorcluster)  [unwired: 9 in, 1 out]
          }
        }
        n230 = event-data("Accepted?"=w633) -> ()  [unwired: 1 in, 1 out]
      }
      event "Exit": Value Change {
        # "Exit the application                                           >> Stop this message generator loop    Cleaning errors if the other loop stop this one"
        n231 = event-data() -> ()  [unwired: 1 in, 1 out]
        n232 = call <vilib>:"Send Local Message.vi"("message queue in"=w657, "message name"="Close", "error in"=w655) -> ("message queue out"=w653:T4, "error out"=w658:errorcluster)  [unwired: 10 in, 1 out]
        n233 = call <vilib>:"Clear Errors.vi"("error in (no error)"=w658) -> ("error out"=w654:errorcluster)  [unwired: 5 in, 1 out]
      }
      event "View": Drag Starting? {
        n234 = event-data() -> ("Data"=w670:T13, "CtlRef"=w672:refnum<vi>, "Coords"=w671:T12)  [unwired: 1 in]
        n235 = invoke class="Tree (strict)" method="Point To Row Column"(reference=w672, error in=w663, "Point"=w671) -> (error out=w662:errorcluster, "Tag"=w669:string)  [unwired: 5 in, 6 out]
        n236 = call <vilib>:"IDtoNode.vi"("error in"=w662, "ID"=w669) -> ("error out"=w661:errorcluster, "invalid Id"=w668:bool, "node ref"=w667:T2)  [unwired: 7 in]
        n237 = case shown="False" w668 {
          tunnel: w667 -> [w680 _]
          tunnel: [w677 TRUE ("Removable")] -> w665
          tunnel: w661 -> [w676 w686]
          tunnel: [w673 w686] -> w660
          frame False {
            n238 = in-place {
              in-place-border: [w683] -> w679
              in-place-border: w676 -> [w682]
              in-place-border: [w681] -> w675
              n239 = in-place-dvr #10(w680) -> (w685:refnum<class "NISE_CEF_Node.lvclass">)  [unwired: 1 out]
              n240 = call-dynamic "EditOptions.vi"("error in"=w682, "node in"=w685) -> ("error out"=w681:errorcluster, "edit options"=w683:T14, "node out"=w684:refnum<class "NISE_CEF_Node.lvclass">)  [unwired: 6 in, 1 out]
              n241 = in-place-dvr #10(w684) -> (w674:errorcluster)  [unwired: 1 out]
            }
            n242 = Unbundle By Name(w679) -> ("movable"=w678:bool)
            n243 = Merge Errors(w674, w675) -> (w673:errorcluster)
            n244 = Not(x=w678) -> (.not. x?=w677:bool)
          }
          frame True {
          }
        }
        n245 = event-data("Data"=w670, "Drag Mode"=enum32{"copy or move", "copy only", "move only"}."move only", "Discard?"=w665) -> ()  [unwired: 1 in, 1 out]
      }
      event "View": Value Change {
        n246 = event-data() -> ("NewVal"=w691:string)  [unwired: 1 in]
        n247 = call <vilib>:"Send Local Message.vi"("message queue in"=w693, "message name"="ActivateNode" ("Message Name"), "message value"=w691, "error in"=w688) -> ("message queue out"=w690:T4, "error out"=w689:errorcluster)  [unwired: 9 in, 1 out]
      }
      event "View": event type 3.0.xa000003a {
        n248 = event-data() -> ("CtlRef"=w702:refnum<vi>, "Coords"=w699:T12)  [unwired: 1 in]
        n249 = invoke class="Tree (strict)" method="Point To Row Column"(reference=w702, error in=w696, "Point"=w699) -> (reference out=w701:refnum<vi>, error out=w695:errorcluster, "Tag"=w700:string)  [unwired: 5 in, 5 out]
        n250 = call <vilib>:"ValidDragDrop.vi"("error in"=w695, "drag over"=w700, "tree ref in"=w701) -> ("error out"=w694:errorcluster, "accepted"=w698:bool)  [unwired: 5 in, 2 out]
        n251 = event-data("Accepted?"=w698) -> ()  [unwired: 1 in, 1 out]
      }
      event Panel Close? {
        # "Intercepts the upper right close panel operation to allow a smooth shutdown as opposed to immediately killing the app."
        n252 = event-data() -> ()  [unwired: 1 in, 1 out]
        n253 = call <vilib>:"Send Local Message.vi"("message queue in"=w707, "message name"="Close?", "error in"=w704) -> ("message queue out"=w705:T4, "error out"=w703:errorcluster)  [unwired: 10 in, 1 out]
        n254 = event-data("Discard?"=TRUE) -> ()  [unwired: 1 in, 1 out]
      }
      event Menu Selection (User) {
        # "#USERCFG It is needed to add a Case for Every item on the menu"
        n255 = event-data() -> ("ItemTag"=w709:string, "ItemPath"=w714:string)  [unwired: 1 in]
        n256 = case shown="\"_File:_New\"" w714 {
          selector: w714 -> [_ _ _ _ _ w744]
          tunnel: w713 -> [w719 w724 w729 w734 w739 w752]
          tunnel: [w715 w720 w725 w730 w735 w749] -> w712
          tunnel: w711 -> [w717 w722 w727 w732 w737 w740]
          tunnel: [w716 w721 w726 w731 w736 w747] -> w710
          tunnel: w709 -> [_ _ _ _ _ w745]
          frame "_File:_New" {
            n257 = call <vilib>:"Send Local Message.vi"("message queue in"=w719, "message name"="New?" ("Message Name"), "error in"=w717) -> ("message queue out"=w715:T4, "error out"=w716:errorcluster)  [unwired: 10 in, 1 out]
          }
          frame "_File:_Open" {
            n258 = call <vilib>:"Send Local Message.vi"("message queue in"=w724, "message name"="Open?" ("Message Name"), "error in"=w722) -> ("message queue out"=w720:T4, "error out"=w721:errorcluster)  [unwired: 10 in, 1 out]
          }
          frame "_File:_Save" {
            n259 = call <vilib>:"Send Local Message.vi"("message queue in"=w729, "message name"="Save" ("Message Name"), "error in"=w727) -> ("message queue out"=w725:T4, "error out"=w726:errorcluster)  [unwired: 10 in, 1 out]
          }
          frame "_File:Save As..." {
            n260 = call <vilib>:"Send Local Message.vi"("message queue in"=w734, "message name"="SaveAs" ("Message Name"), "error in"=w732) -> ("message queue out"=w730:T4, "error out"=w731:errorcluster)  [unwired: 10 in, 1 out]
          }
          frame "_File:_Exit" {
            n261 = call <vilib>:"Send Local Message.vi"("message queue in"=w739, "message name"="Close?" ("Message Name"), "error in"=w737) -> ("message queue out"=w735:T4, "error out"=w736:errorcluster)  [unwired: 10 in, 1 out]
          }
          frame Default {
            n262 = Bundle("ItemTag"=w745, w744) -> (w743:cluster{"ItemTag":string, string})  [unwired: 1 in]
            n263 = Flatten To String(anything=w743, error in (no error)=w740) -> (data string=w742:string, error out=w741:errorcluster)  [unwired: 2 in, 1 out]
            n264 = call <vilib>:"Send Local Message.vi"("message queue in"=w752, "message name"="CleansubPanel", "error in"=w741) -> ("message queue out"=w751:T4, "error out"=w748:errorcluster)  [unwired: 10 in, 1 out]
            n265 = call <vilib>:"Send Local Message.vi"("message queue in"=w751, "message name"="CustomFileMenu" ("Message Name"), "message value"=w742, "error in"=w748) -> ("message queue out"=w749:T4, "error out"=w747:errorcluster)  [unwired: 9 in, 1 out]
          }
        }
      }
    }
    n266 = call "Error.vi"("error in (no error)"=w537, "message queue in"=w538) -> ()  [unwired: 9 in, 1 out]
  }
